vi "IntakeRefSelector.vi"(10 "Enum 2":T1) -> (2 "String":string="FrontRightIntakeMotor")   [LabVIEW 2014, in "IntakeLib.lvlib"]
uses:
  IntakeLib.lvlib
  IntakeRefs.ctl
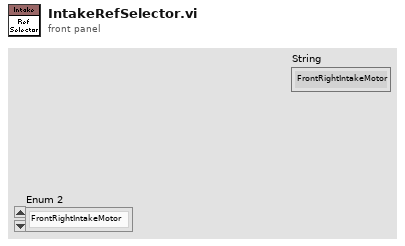
[diagram p1: front panel]
types:
  T1 = typedef "IntakeLib.lvlib/IntakeRefs.ctl" = enum16{"FrontRightIntakeMotor", "FrontLeftIntakeMotor", "BackLeftIntakeMotor", "BackRightIntakeMotor", "IntakeCyl"}
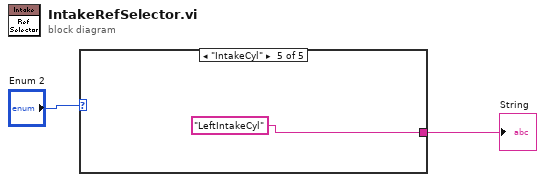
[diagram p0: block diagram]
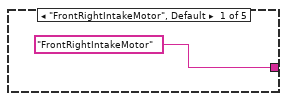
[diagram p2: hidden frame]
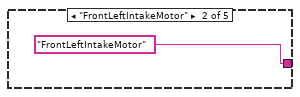
[diagram p3: hidden frame]
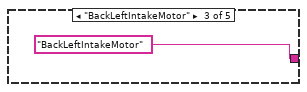
[diagram p4: hidden frame]
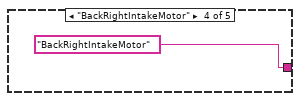
[diagram p5: hidden frame]
diagram:
  n1 = case shown="\"IntakeCyl\"" "Enum 2" {
    tunnel: ["FrontRightIntakeMotor" "FrontLeftIntakeMotor" "BackLeftIntakeMotor" "BackRightIntakeMotor" "LeftIntakeCyl"] -> w1
    frame "FrontRightIntakeMotor", Default {
    }
    frame "FrontLeftIntakeMotor" {
    }
    frame "BackLeftIntakeMotor" {
    }
    frame "BackRightIntakeMotor" {
    }
    frame "IntakeCyl" {
    }
  }
  "String" <- w1
